vi "Unpack I32.vi"(11 "Broadcast I32 Msg In":refnum<class "Broadcast I32 Msg.lvclass">) -> (2 "Value":i32, 3 "Name":string)   [LabVIEW 2015, in "IViewable.lvlib" / "Broadcast I32 Msg.lvclass"]
uses:
  Broadcast I32 Msg.lvclass
  Broadcast I32 Msg.lvclass/Broadcast I32 Msg.ctl
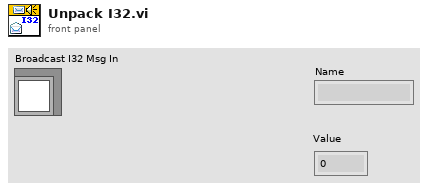
[diagram p1: front panel]
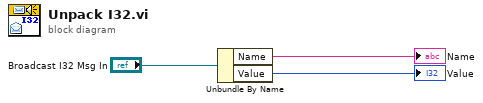
[diagram p0: block diagram]
diagram:
  n1 = Unbundle By Name("Broadcast I32 Msg In") -> ("Name"=→"Name":string, "Value"=→"Value":i32)
